vi "FTW-PerfTest-CompileTime.vi"() -> (0 "Test Result":errorcluster)   [LabVIEW 2015]
panel:
  out "Compile Times":T1(graph)={"[0]"=5.84790307818912, "[1]"=4.014325281692436, "[2]"=1.413922252948396, "[3]"=1.214117234951118}
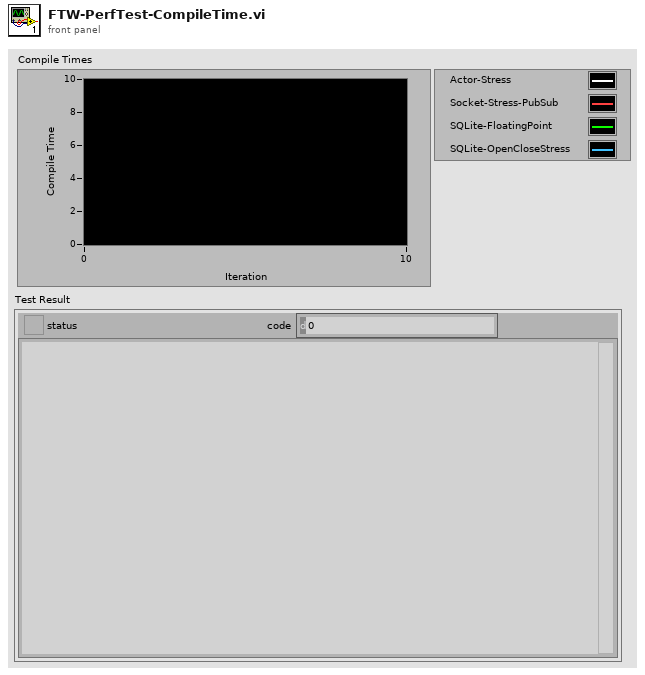
[diagram p1: front panel]
types:
  T1 = cluster{"[0]":dbl, "[1]":dbl, "[2]":dbl, "[3]":dbl}
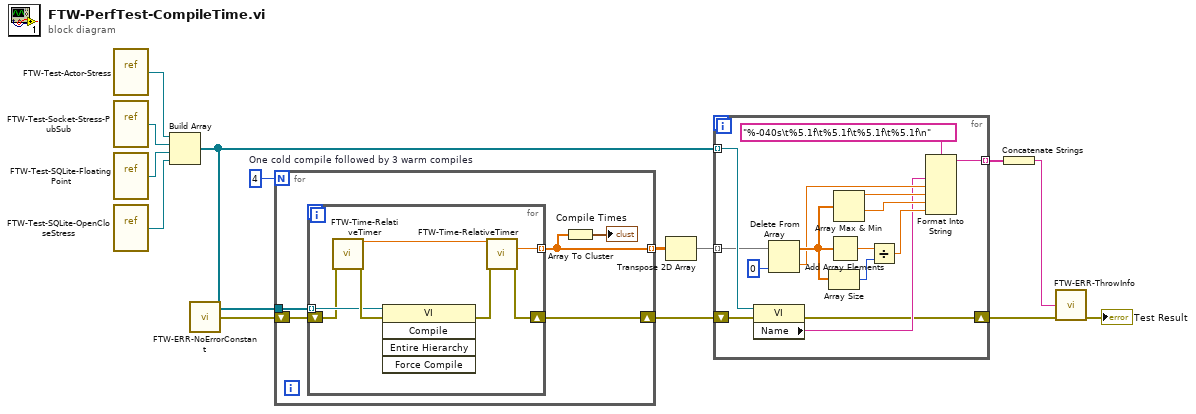
[diagram p0: block diagram]
diagram:
  w7 = 4  # One cold compile followed by 3 warm compiles
  n1 = vi-ref "FTW-Test-Actor-Stress.vi"() -> (w14:refnum<vi>)
  n2 = vi-ref "FTW-Test-Socket-Stress-PubSub.vi"() -> (w13:refnum<vi>)
  n3 = vi-ref "FTW-Test-SQLite-FloatingPoint.vi"() -> (w12:refnum<vi>)
  n4 = vi-ref "FTW-Test-SQLite-OpenCloseStress.vi"() -> (w11:refnum<vi>)
  n5 = Build Array(w14, w13, w12, w11) -> (w5:refnum<vi>[])
  n6 = call "FTW-ERR-NoErrorConstant.vi"() -> ("no error"=w10:errorcluster)
  n7 = for {
    N: w7 -> [_]
    tunnel: w5 -> [w19]
    shift-right: [w15] -> w3
    shift-left: w10 -> [w18]
    tunnel: [w16] -> w6 mode=indexing
    n8 = for {
      shift-right: [w21] -> w15
      shift-left: w18 -> [w22]
      tunnel: [w20] -> w16 mode=indexing
      tunnel: w19 -> [w23] mode=indexing
      n9 = call "FTW-Time-RelativeTimer.vi"("error in"=w22) -> ("Current Timer Value"=w24:dbl, "error out"=w26:errorcluster)  [unwired: 12 in, 1 out]
      n10 = invoke class="VI" method="Compile"(reference=w23, error in=w26) -> (error out=w25:errorcluster)  [unwired: 3 in, 4 out]
      n11 = call "FTW-Time-RelativeTimer.vi"("Previous Timer Value"=w24, "error in"=w25) -> ("Elapsed Time"=w20:dbl, "error out"=w21:errorcluster)  [unwired: 11 in, 1 out]
    }
    n12 = Array To Cluster(array=w16) -> (cluster=→"Compile Times":T1)
  }
  n13 = Transpose 2D Array(2D array=w6) -> (transposed array=w4:dbl[][])
  n14 = for {
    tunnel: w4 -> [w27] mode=indexing
    tunnel: w5 -> [w31] mode=indexing
    shift-right: [w29] -> w1
    shift-left: w3 -> [w30]
    tunnel: [w28] -> w2 mode=indexing
    n15 = property class="VI"(reference=w31, error in=w30) -> (error out=w29:errorcluster, "Name"=w35:string)  [unwired: 1 out]
    n16 = Delete From Array(array=w27, index=0) -> (deleted portion=w37:dbl, array with subset deleted=w38:dbl[])  [unwired: 1 in]
    n17 = Array Size(array=w38) -> (size(s)=w34:i32)
    n18 = Add Array Elements(numeric array=w38) -> (sum=w33:dbl)
    n19 = Array Max & Min(array=w38) -> (max value=w39:dbl, min value=w40:dbl)  [unwired: 2 out]
    n20 = Divide(x=w33, y=w34) -> (x/y=w41:dbl)
    n21 = Format Into String(format string="%-040s\t%5.1f\t%5.1f\t%5.1f\t%5.1f\n", w35, w37, w39, w40, w41) -> (resulting string=w28:string)  [unwired: 2 in, 1 out]
  }
  n22 = Concatenate Strings(w2) -> (w9:string)
  n23 = call "FTW-ERR-ThrowInfo.vi"("Informational Message"=w9, "error in"=w1) -> ("error out"=→"Test Result":errorcluster)  [unwired: 13 in]
